vi "subVI1.vi"(11 "Numeric":dbl) -> (2 "B":bool, 3 "A":bool, 8 "x/y":dbl)   [LabVIEW 2020]
panel:
  out "-1, 0, 1":i64
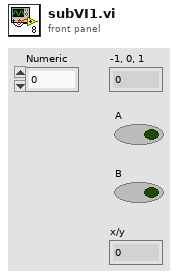
[diagram p1: front panel]
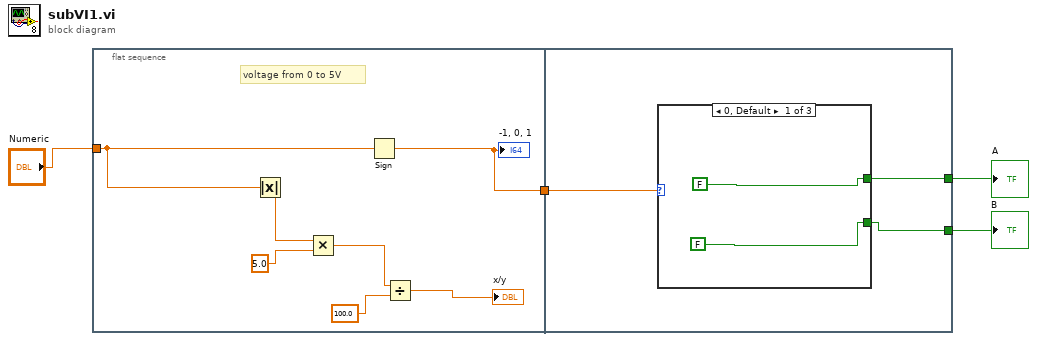
[diagram p0: block diagram]
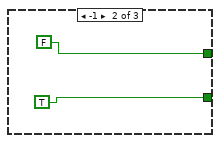
[diagram p2: hidden frame]
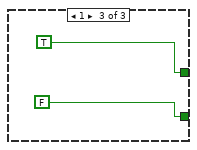
[diagram p3: hidden frame]
diagram:
  n1 = flat-sequence {
    tunnel: "Numeric" -> [w6]
    tunnel: [w5] -> w4
    tunnel: [w14] -> w2
    tunnel: [w13] -> w3
    tunnel: w4 -> [w12]
    frame #0 {
      # "voltage from 0 to 5V"
      n2 = Absolute Value(x=w6) -> (abs(x)=w11:dbl)
      n3 = Multiply(x=w11, y=5.0) -> (x*y=w10:dbl)
      n4 = Sign(1:w6) -> (0:w5:dbl)
      "-1, 0, 1" <- w5
      n5 = Divide(x=w10, y=100.0) -> (x/y=→"x/y":dbl)
    }
    frame #1 {
      n6 = case shown="0, Default" w12 {
        tunnel: [FALSE FALSE TRUE] -> w14
        tunnel: [FALSE TRUE FALSE] -> w13
        frame 0, Default {
        }
        frame -1 {
        }
        frame 1 {
        }
      }
    }
  }
  "B" <- w3
  "A" <- w2
